vi "SubVI-AOMvolt-Power Calibration for 1064-v5.vi"(0 "Min voltage (V)":dbl=0.5, 2 "Max voltage (V)":dbl=4.5, 3 "scan step #":dbl=25.0, 5 "milliseconds to wait":u32=200) -> (6 "output cluster":T1, 7 "Polynomial Coefficients":dbl[](array[numeric]) format="%0.2f")   [LabVIEW 2014]
uses:
  Main-Stage-Based/(Global) Current handle and LaserPower_YCC.vi
  <vilib>/Utility/file.llb/Write To Spreadsheet File (DBL).vi
  <vilib>/Analysis/NI_AALPro.lvlib
panel:
  out "Cal-Power (mW)":dbl[](array[numeric])
  out "Cal-AOM (V)":dbl[](array[numeric])
  out "Power-AOM Graph":T2(graph)
  out "Voltage to AOM (V)":dbl
  out "Power readout (mW)":dbl
  out "Scan size per step (V)":dbl=0.25
  in  "save cal curve?":bool
  # "**activate \ncontinuous power\ncontinuous AOM"
  # "continuous scaning power \nover AOM voltage range"
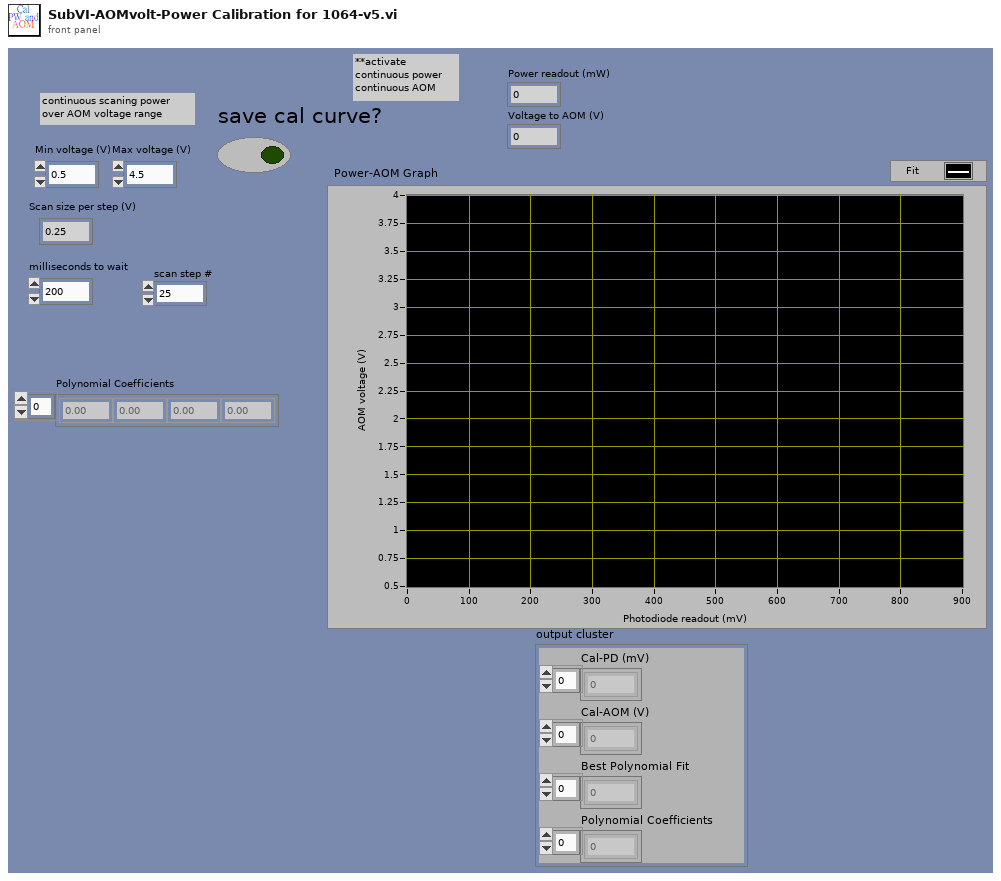
[diagram p1: front panel]
types:
  T1 = cluster{"Cal-PD (mV)":dbl[], "Cal-AOM (V)":dbl[], "Best Polynomial Fit":dbl[], "Polynomial Coefficients":dbl[]}
  T2 = cluster{"Cal-PD (mV)":dbl[], "Cal-AOM (V)":dbl[]}[]
  T3 = cluster{"Cal-Power (mW)":dbl[], "Best Polynomial Fit":dbl[]}
  T4 = cluster{"Cal-Power (mW)":dbl[], "Cal-AOM (V)":dbl[]}
  T5 = cluster{"Cal-Power (mW)":dbl[], "Cal-AOM (V)":dbl[], "Best Polynomial Fit":dbl[], "Polynomial Coefficients":dbl[]}
  T6 = cluster{"Cal-Power (mW)":dbl[], "Cal-AOM (V)":dbl[]}[]
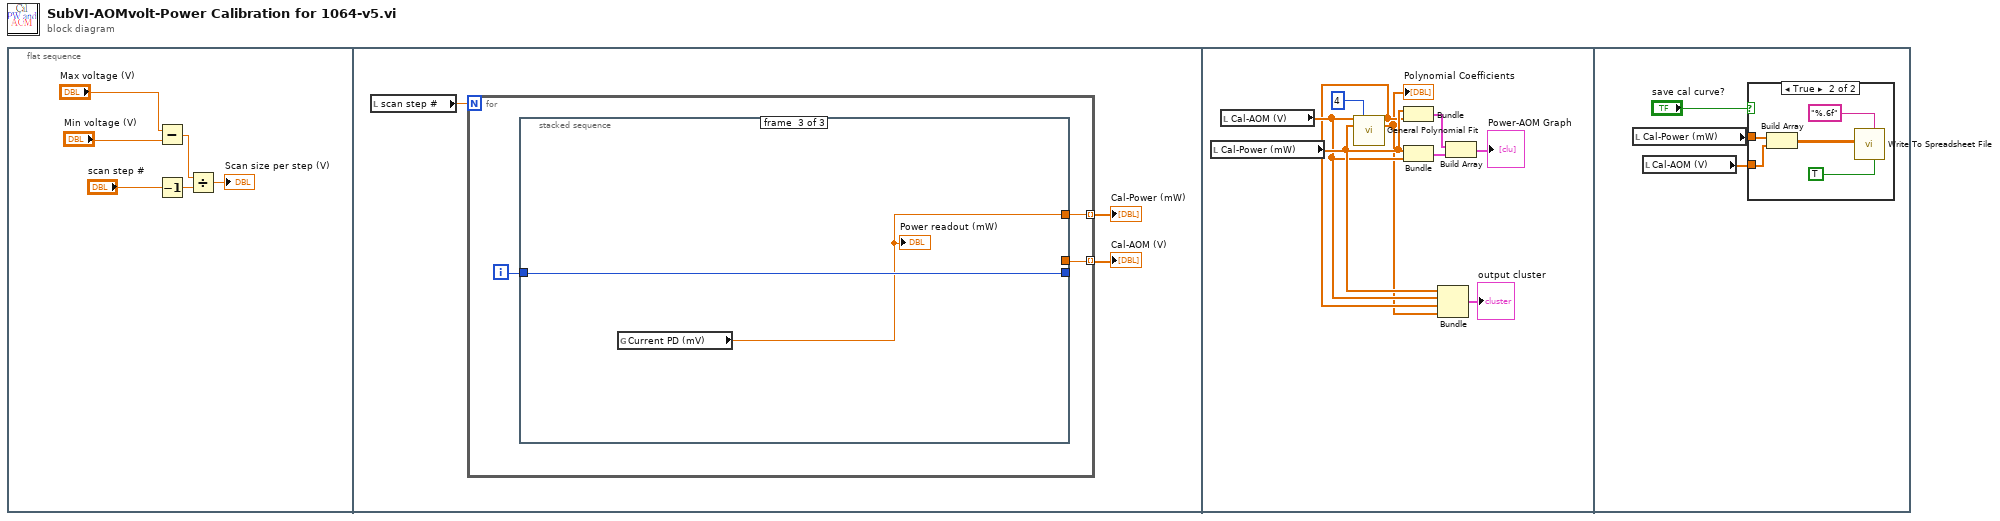
[diagram p0: block diagram]
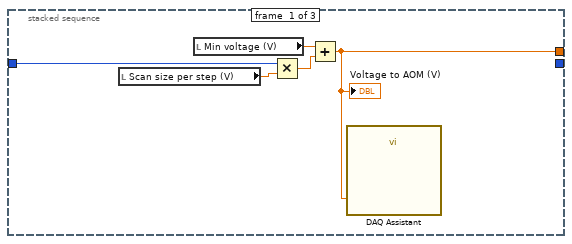
[diagram p2: hidden frame]
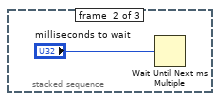
[diagram p3: hidden frame]
diagram:
  n1 = flat-sequence {
    frame #0 {
      n2 = Subtract(x="Max voltage (V)", y="Min voltage (V)") -> (x-y=w3:dbl)
      n3 = Decrement(x="scan step #") -> (x-1=w5:dbl)
      n4 = Divide(x=w3, y=w5) -> (x/y=→"Scan size per step (V)":dbl)
    }
    frame #1 {
      n5 = local read "scan step #"() -> (w9:dbl)
      n6 = for {
        N: w9 -> [_]
        tunnel: [w11] -> w7 mode=indexing
        tunnel: [w10] -> w8 mode=indexing
        i -> [w12]
        n7 = stacked-sequence {
          tunnel: w12 -> [w14 _ w20]
          tunnel: [_ _ w20] -> _
          tunnel: [_ _ w19] -> w11
          tunnel: [w17 _ _] -> w10
          frame #0 {
            n8 = local read "Scan size per step (V)"() -> (w15:dbl)
            n9 = local read "Min voltage (V)"() -> (w16:dbl)
            n10 = Multiply(x=w14, y=w15) -> (x*y=w13:dbl)
            n11 = Add(x=w16, y=w13) -> (x+y=w17:dbl)
            "Voltage to AOM (V)" <- w17
            n12 = call "DAQ Assistant"("data"=w17) -> ()  [unwired: 17 in, 2 out]
          }
          frame #1 {
            n13 = Wait Until Next ms Multiple(millisecond multiple="milliseconds to wait") -> ()  [unwired: 1 out]
          }
          frame #2 {
            n14 = global read "(Global) Current handle and LaserPower_YCC.vi" "Current PD (mV)"() -> (w19:dbl)
            "Power readout (mW)" <- w19
          }
        }
      }
      "Cal-AOM (V)" <- w8
      "Cal-Power (mW)" <- w7
    }
    frame #2 {
      n15 = local read "Cal-Power (mW)"() -> (w25:dbl[])
      n16 = local read "Cal-AOM (V)"() -> (w24:dbl[])
      n17 = call <vilib>:"General Polynomial Fit.vi"("Y"=w24, "polynomial order"=4, "X"=w25) -> ("Best Polynomial Fit"=w23:dbl[], "Polynomial Coefficients"=w22:dbl[])  [unwired: 9 in, 2 out]
      "Polynomial Coefficients" <- w22
      n18 = Bundle("Cal-Power (mW)"=w25, "Best Polynomial Fit"=w23) -> (w28:T3)  [unwired: 1 in]
      n19 = Bundle("Cal-Power (mW)"=w25, "Cal-AOM (V)"=w24) -> (w27:T4)  [unwired: 1 in]
      n20 = Bundle("Cal-Power (mW)"=w25, "Cal-AOM (V)"=w24, "Best Polynomial Fit"=w23, "Polynomial Coefficients"=w22) -> (→"output cluster":T5)  [unwired: 1 in]
      n21 = Build Array(w28, w27) -> (→"Power-AOM Graph":T6)
    }
    frame #3 {
      n22 = local read "Cal-Power (mW)"() -> (w31:dbl[])
      n23 = local read "Cal-AOM (V)"() -> (w30:dbl[])
      n24 = case shown="True" "save cal curve?" {
        tunnel: w31 -> [_ w36]
        tunnel: w30 -> [_ w35]
        frame False {
        }
        frame True {
          n25 = Build Array(w36, w35) -> (w34:dbl[][])
          n26 = call-poly <vilib>:"Write To Spreadsheet File.vi"("transpose? (no:F)"=TRUE, "format (%.3f)"="%.6f", "2D data"=w34) -> ()  [unwired: 3 in, 3 out]
        }
      }
    }
  }
